vi "Size of Data Type.vi"(11 "Data Type":T1=1 items=["unknown", "BOOLEAN", "INTEGER8", "INTEGER16", "INTEGER32", "UNSIGNED8", "UNSIGNED16", "UNSIGNED32", "REAL32", "VISIBLE_STRING", "OCTET_STRING", "UNICODE_STRING", "TIME_OF_DAY", "TIME_DIFFERENCE", "RESERVED1", "DOMAIN", "INTEGER24", "REAL64", "INTEGER40", "INTEGER48", "INTEGER56", "INTEGER64", "UNSIGNED24", "RESERVED2", "UNSIGNED40", "UNSIGNED48", "UNSIGNED56", "UNSIGNED64", "RESERVED3", "RESERVED4", "RESERVED5", "RESERVED6", "PDO_COMMUNICATION_PARAMETER", "PDO_MAPPING", "SDO_PARAMETER", "IDENTITY", "RESERVED7"]) -> (3 "Size":u8 format="%d Bits")   [LabVIEW 2020, in "CANopen.lvlib"]
uses:
  CANopen.lvlib
  Typedefs/Data Type.ctl
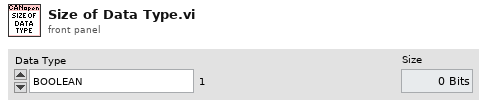
[diagram p1: front panel]
types:
  T1 = typedef "CANopen.lvlib/Data Type.ctl" = u16
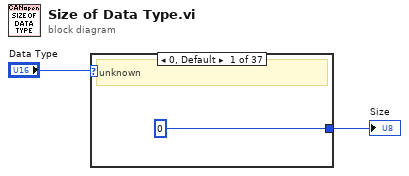
[diagram p0: block diagram]
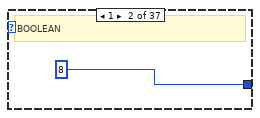
[diagram p2: hidden frame]
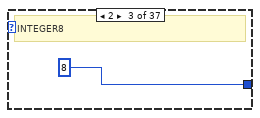
[diagram p3: hidden frame]
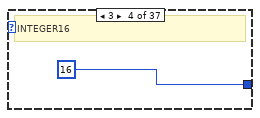
[diagram p4: hidden frame]
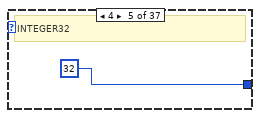
[diagram p5: hidden frame]
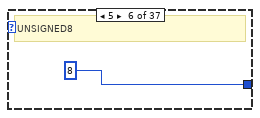
[diagram p6: hidden frame]
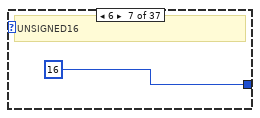
[diagram p7: hidden frame]
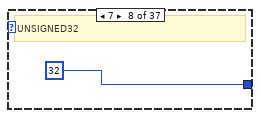
[diagram p8: hidden frame]
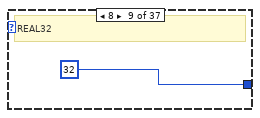
[diagram p9: hidden frame]
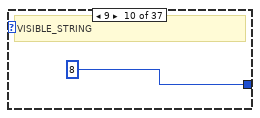
[diagram p10: hidden frame]
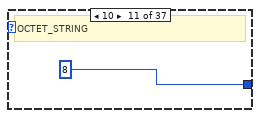
[diagram p11: hidden frame]
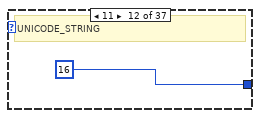
[diagram p12: hidden frame]
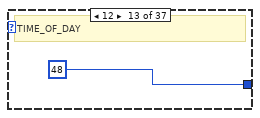
[diagram p13: hidden frame]
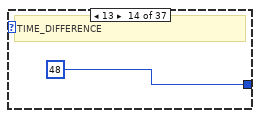
[diagram p14: hidden frame]
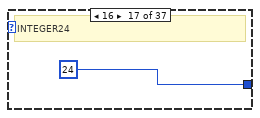
[diagram p17: hidden frame]
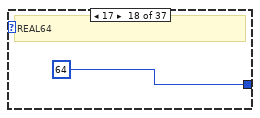
[diagram p18: hidden frame]
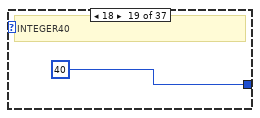
[diagram p19: hidden frame]
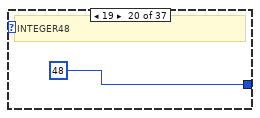
[diagram p20: hidden frame]
diagram:
  n1 = case shown="0, Default" "Data Type" {
    tunnel: [u8 0 u8 8 u8 8 u8 16 u8 32 u8 8 u8 16 u8 32 u8 32 u8 8 u8 8 u8 16 u8 48 u8 48 _ _ u8 24 u8 64 u8 40 u8 48 u8 56 u8 64 u8 24 _ u8 40 u8 48 u8 56 u8 64 _ _ _ _ u8 96 _ _ u8 136 _] -> w1
    frame 0, Default {
      # "unknown"
    }
    frame 1 {
      # "BOOLEAN"
    }
    frame 2 {
      # "INTEGER8"
    }
    frame 3 {
      # "INTEGER16"
    }
    frame 4 {
      # "INTEGER32"
    }
    frame 5 {
      # "UNSIGNED8"
    }
    frame 6 {
      # "UNSIGNED16"
    }
    frame 7 {
      # "UNSIGNED32"
    }
    frame 8 {
      # "REAL32"
    }
    frame 9 {
      # "VISIBLE_STRING"
    }
    frame 10 {
      # "OCTET_STRING"
    }
    frame 11 {
      # "UNICODE_STRING"
    }
    frame 12 {
      # "TIME_OF_DAY"
    }
    frame 13 {
      # "TIME_DIFFERENCE"
    }
    frame 14 {
      # "RESERVED1"
    }
    frame 15 {
      # "DOMAIN"
    }
    frame 16 {
      # "INTEGER24"
    }
    frame 17 {
      # "REAL64"
    }
    frame 18 {
      # "INTEGER40"
    }
    frame 19 {
      # "INTEGER48"
    }
    frame 20 {
      # "INTEGER56"
    }
    frame 21 {
      # "INTEGER64"
    }
    frame 22 {
      # "UNSIGNED24"
    }
    frame 23 {
      # "RESERVED2"
    }
    frame 24 {
      # "UNSIGNED40"
    }
    frame 25 {
      # "UNSIGNED48"
    }
    frame 26 {
      # "UNSIGNED56"
    }
    frame 27 {
      # "UNSIGNED64"
    }
    frame 28 {
      # "RESERVED3"
    }
    frame 29 {
      # "RESERVED4"
    }
    frame 30 {
      # "RESERVED5"
    }
    frame 31 {
      # "RESERVED6"
    }
    frame 32 {
      # "PDO_COMMUNICATION_PARAMETER"
    }
    frame 33 {
      # "PDO_MAPPING"
    }
    frame 34 {
      # "SDO_PARAMETER"
    }
    frame 35 {
      # "IDENTITY"
    }
    frame 36 {
      # "RESERVED7"
    }
  }
  "Size" <- w1
